vi "Handle Project Copy Cleanup.vi"(8 "error in (no error)":errorcluster, 9 "More Scripting?":bool, 10 "Target Path":path, 11 "Project in":refnum<vi>) -> ()   [LabVIEW 2016, in "NI_NPW_Project Copying.lvlib"]
uses:
  <resource>/dialog/NewProjectWizard/Project Copying/NI_NPW_Project Copying.lvlib
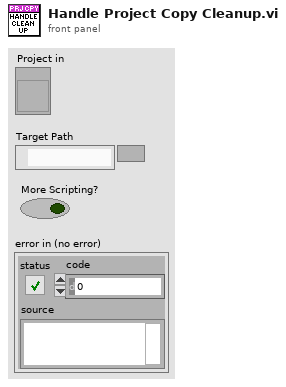
[diagram p1: front panel]
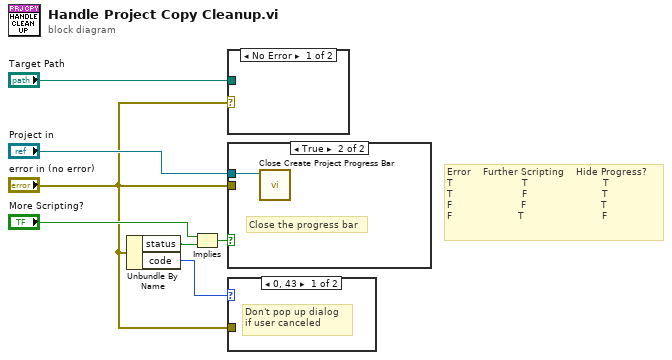
[diagram p0: block diagram]
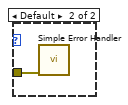
[diagram p2: hidden frame]
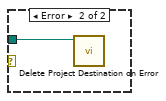
[diagram p3: hidden frame]
diagram:
  # "Error    Further Scripting    Hide Progress?\nT                       T                         T\nT                       F                         T\nF                       F                         T\nF                      T                          F"
  n1 = Unbundle By Name("error in (no error)") -> ("status"=w4:bool, "code"=w2:i32)
  n2 = Implies(1:w4, 2:"More Scripting?") -> (0:w5:bool)
  n3 = case shown="No Error" "error in (no error)" {
    tunnel: "Target Path" -> [_ w8]
    frame No Error {
    }
    frame Error {
      n4 = call <resource>:"Delete Project Destination on Error.vi"("Project Destination Root"=w8) -> ()  [unwired: 11 in]
    }
  }
  n5 = case shown="True" w5 {
    tunnel: "Project in" -> [_ w9]
    tunnel: "error in (no error)" -> [_ _]
    frame False {
      # "Don't close the progress bar...more scripting is about to happen"
    }
    frame True {
      # "Close the progress bar"
      n6 = call <resource>:"Close Create Project Progress Bar.vi"("Project"=w9) -> ()  [unwired: 9 in, 2 out]
    }
  }
  n7 = case shown="0, 43" w2 {
    tunnel: "error in (no error)" -> [_ w10]
    frame 0, 43 {
      # "Don't pop up dialog\nif user canceled"
    }
    frame Default {
      n8 = call <vilib>:"Simple Error Handler.vi"("error in (no error)"=w10) -> ()  [unwired: 4 in, 5 out]
    }
  }
